vi "SMO.Example.GetPublicEvents.vi"(8 "error in (no error)":errorcluster, 11 "SMO.Example":refnum<class "SMO.Example.lvclass">) -> (0 "error out":errorcluster, 1 "Dependency Events":refnum<user-event>, 2 "SMO.Example Public Events":T1, 3 "SMO.Example out":refnum<class "SMO.Example.lvclass">)   [LabVIEW 2013, in "SMO.Example.lvclass"]
doc: "---------------------------------------------------------------\nJKI State Machine Objects™\nhttp://jki.net/state-machine-objects/\nCopyright (C) 2005-2015, JKI <info@jki.net>\nALL RIGHTS RESERVED"
uses:
  SMO.Example.lvclass
  Typedefs/PublicEvents--Cluster.ctl
  Typedefs/DataChanged--EventData--Cluster.ctl
  src/SMO/Typedefs/SMO Dependency Event--Cluster.ctl
  src/SMO/Typedefs/SMO Dependency Event--Enum.ctl
  SMO.Example.lvclass/SMO.Example.ctl
  src/SMO/SMO.lvclass
panel:
  # "For instructions on how to use the JKI State Machine Objects, examples and video tutorials, visit:\nhttp://jki.net/state-machine-objects/\n\nJKI State Machine Objects™\nhttp://jki.net/state-machine-objects/\nCopyright (C) 2005-2015, JKI <info@jki.net>\nALL RIGHTS RESERVED"
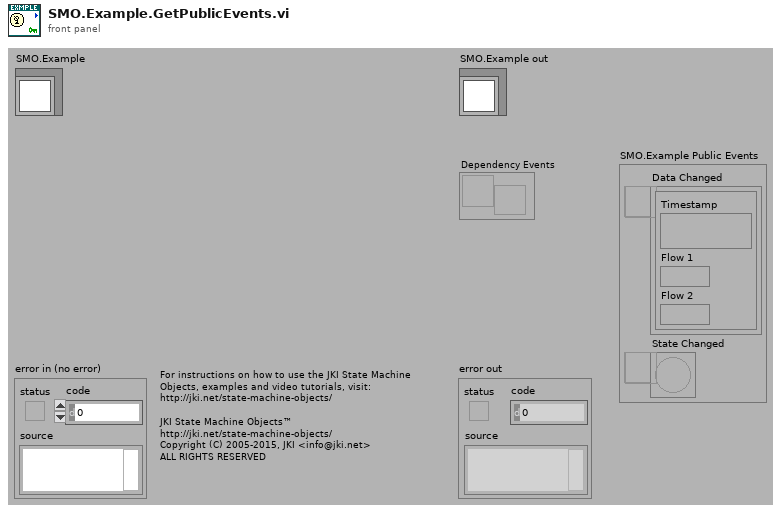
[diagram p1: front panel]
types:
  T1 = typedef "SMO.Example.lvclass/PublicEvents--Cluster.ctl" = cluster{"Data Changed":refnum<user-event>, "State Changed":refnum<user-event>}
  T2 = typedef "SMO.Example.lvclass/PrivateData--Ref.ctl" = refnum<data-value>
  T3 = typedef "SMO.Example.lvclass/PrivateData--Cluster.ctl" = cluster{"Configuration":T4, "Public Events":T1, "Protected Events":T5, "Flow 1":dbl, "Flow 2":dbl}
  T4 = typedef "SMO.Example.lvclass/Configuration--Cluster.ctl" = cluster{"Suffix":string}
  T5 = typedef "SMO.Example.lvclass/ProtectedEvents--Cluster.ctl" = cluster{"API_Template":refnum<user-event>, "PumpState":refnum<user-event>, "Valve State":refnum<user-event>}
  T6 = typedef "SMO.lvclass/Protected Events.ctl" = cluster{"StopProcesses":refnum<user-event>, "AbortProcesses":refnum<user-event>, "Config Changed":refnum<user-event>, "Dependency":refnum<user-event>}
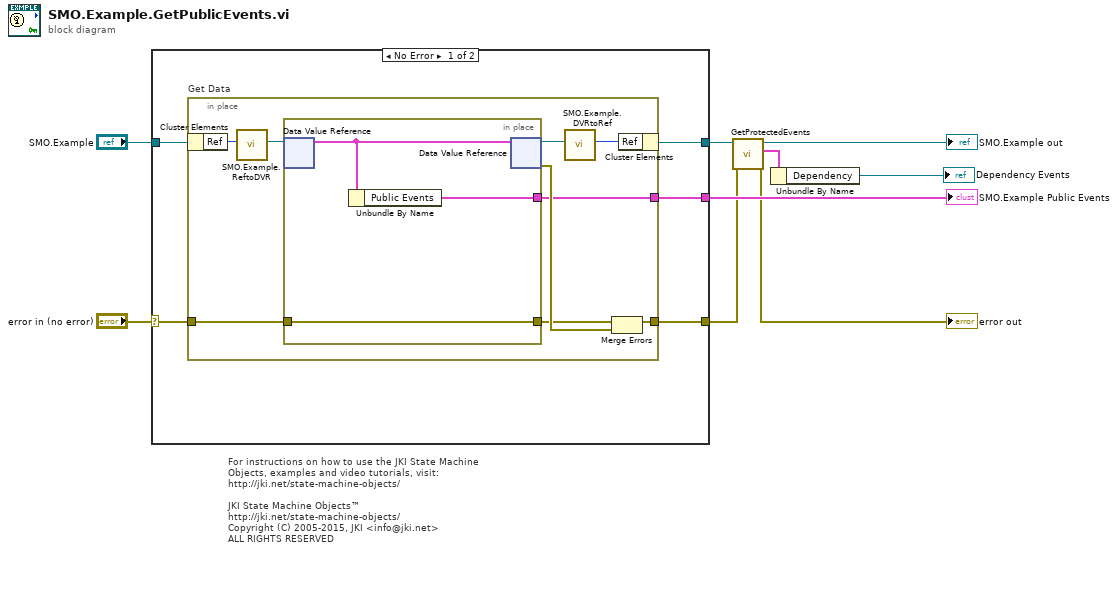
[diagram p0: block diagram]
diagram:
  # "For instructions on how to use the JKI State Machine Objects, examples and video tutorials, visit:\nhttp://jki.net/state-machine-objects/\n\nJKI State Machine Objects™\nhttp://jki.net/state-machine-objects/\nCopyright (C) 2005-2015, JKI <info@jki.net>\nALL RIGHTS RESERVED"
  n1 = case shown="No Error" "error in (no error)" {
    selector: "error in (no error)" -> [w13 w27]
    tunnel: "SMO.Example" -> [w14 w28]
    tunnel: [w12 w27] -> w3
    tunnel: [w11 w28] -> w6
    tunnel: [w10 _] -> w5
    frame No Error {
      n2 = in-place "Get Data" {
        in-place-border: w13 -> [w23]
        in-place-border: [w20] -> w12
        in-place-border: [w19] -> w10
        n3 = in-place-cluster #1(w14) -> ("Ref"=w18:u32)
        n4 = call "SMO.Example.ReftoDVR.vi"("Ref"=w18) -> ("Ref"=w17:T2)  [unwired: 10 in]
        n5 = in-place {
          in-place-border: w23 -> [w25]
          in-place-border: [w25] -> w21
          in-place-border: [w24] -> w19
          n6 = in-place-dvr #2(w17) -> (w26:T3)  [unwired: 1 out]
          n7 = Unbundle By Name(w26) -> ("Public Events"=w24:T1)
          n8 = in-place-dvr #2(w26) -> (w16:T2, w22:errorcluster)
        }
        n9 = call "SMO.Example.DVRtoRef.vi"("Ref"=w16) -> ("Ref"=w15:u32)  [unwired: 10 in]
        n10 = Merge Errors(w21, w22) -> (w20:errorcluster)
        n11 = in-place-cluster #1("Ref"=w15) -> (w11:refnum<class "SMO.Example.lvclass">)
      }
    }
    frame Error {
    }
  }
  "SMO.Example Public Events" <- w5
  n12 = call "GetProtectedEvents.vi"("error in (no error)"=w3, "SMO"=w6) -> ("error out"=→"error out":errorcluster, "SMO Protected Events"=w2:T6, "SMO out"=→"SMO.Example out":refnum<class "SMO.Example.lvclass">)  [unwired: 7 in]
  n13 = Unbundle By Name(w2) -> ("Dependency"=→"Dependency Events":refnum<user-event>)
